vi "Test Build Path Multi-OS.vi"() -> (0 "error out":errorcluster, 3 "Pass":bool)   [LabVIEW 2021]
uses:
  File_CIF_U.lvlib
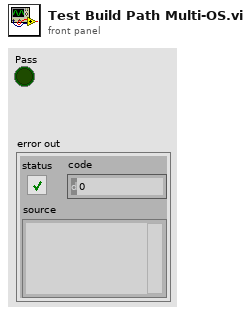
[diagram p1: front panel]
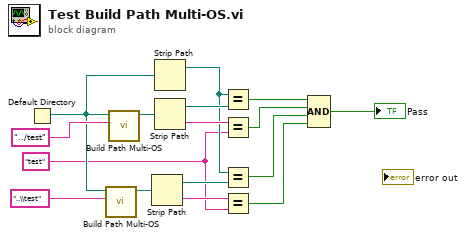
[diagram p0: block diagram]
diagram:
  w3 = "test" ("name or relative path")
  n1 = Default Directory() -> (w8:path)
  n2 = call "Build Path Multi-OS.vi"("name or relative path"="..\\test", "base path"=w8) -> ("appended path"=w9:path)  [unwired: 9 in]
  n3 = call "Build Path Multi-OS.vi"("name or relative path"="../test", "base path"=w8) -> ("appended path"=w15:path)  [unwired: 9 in]
  n4 = Strip Path(path=w9) -> (stripped path=w6:path, name=w5:string)
  n5 = Strip Path(path=w8) -> (stripped path=w4:path)  [unwired: 1 out]
  n6 = Strip Path(path=w15) -> (stripped path=w14:path, name=w13:string)
  n7 = Equal?(x=w4, y=w14) -> (x = y?=w12:bool)
  n8 = Equal?(x=w13, y=w3) -> (x = y?=w11:bool)
  n9 = Equal?(x=w4, y=w6) -> (x = y?=w2:bool)
  n10 = Equal?(x=w5, y=w3) -> (x = y?=w1:bool)
  n11 = Compound Arithmetic op=AND(w12, w11, w2, w1) -> (→"Pass":bool)
